vi "05_orezani_signalu_na_celistve_periody.vi"() -> ()   [LabVIEW 2019]
uses:
  <vilib>/Analysis/baseanly.llb/Mean (DBL).vi
  <vilib>/measure/NI_MABase.lvlib
  <vilib>/Analysis/NI_AALBase.lvlib
panel:
  out "Pouze kompletni periody":waveform(dbl)(graph)={"t0"=timestamp(0 s since 1904-01-01), "dt"=0.001, "Y"=array[484 elements]}
  out "Delka signalu celych period":dbl=0.4981312127236578
  out "Pocet celistvych period":dbl=30.0
  out "Necelistvy pocet period?":bool=TRUE
  out "Delka celeho signalu (s)":dbl=0.5
  out "Pocet period":dbl=30.112547892720322
  out "Prumerna perioda signalu(s)":dbl=0.01660437375745526
  out "Prumerna frekvence (Hz)":dbl=60.22509578544064 format="%0.2f"
  in  "Cas necitlivosti (s)":dbl=0.005
  out "Pole casu pruchodu nulou":dbl[](array[numeric])=[0.009000000000000001, 0.017, 0.025, 0.034, 0.042, 0.05, 0.059000000000000004, 0.067, 0.075, 0.084, 0.092, 0.1, 0.109, 0.117, 0.125, 0.134, 0.14200000000000002, 0.15, 0.159, 0.167, 0.17500000000000002, 0.184, 0.192, 0.2, 0.209, 0.217, 0.225, 0.234, 0.242, 0.25, 0.259, 0.267, 0.275, 0.28400000000000003, 0.292, 0.3, 0.309, 0.317, 0.325, 0.334, 0.342, 0.35000000000000003, 0.359, 0.367, 0.375, 0.384, 0.392, 0.4, 0.40900000000000003, 0.417, 0.425, 0.434, 0.442, 0.45, 0.459, 0.467, 0.47500000000000003, 0.484, 0.492]
  out "Originalni signal":waveform(dbl)(graph)={"t0"=timestamp(0 s since 1904-01-01), "dt"=0.001, "Y"=array[500 elements]}
  out "dt (s)":dbl=0.001
  out "Vzorkovaci Frekvence (N)":dbl=1000.0
  in  "Amplituda sumu":dbl format="%.2p"
  in  "Info o vzorkovani":T1={"Vzorkovaci frekvence"=1000.0, "Pocet vzorku v okne"=500.0} {"Vzorkovaci frekvence" format="%.2p"}
  in  "Faze":dbl format="%.2p"
  in  "Amplituda":dbl=10.0 format="%0.2p"
  in  "Frekvence":dbl=60.000000000000604 format="%0.2p"
  # "Jak budete zvedat frekvenci signalu, sledujte, ze mezera mezi nulou a poslednim vzorkem se meni, jelikoz samotna 1 perioda ma\nmene vzorku. Zkuste menit aj vzorkovaci frekvenci."
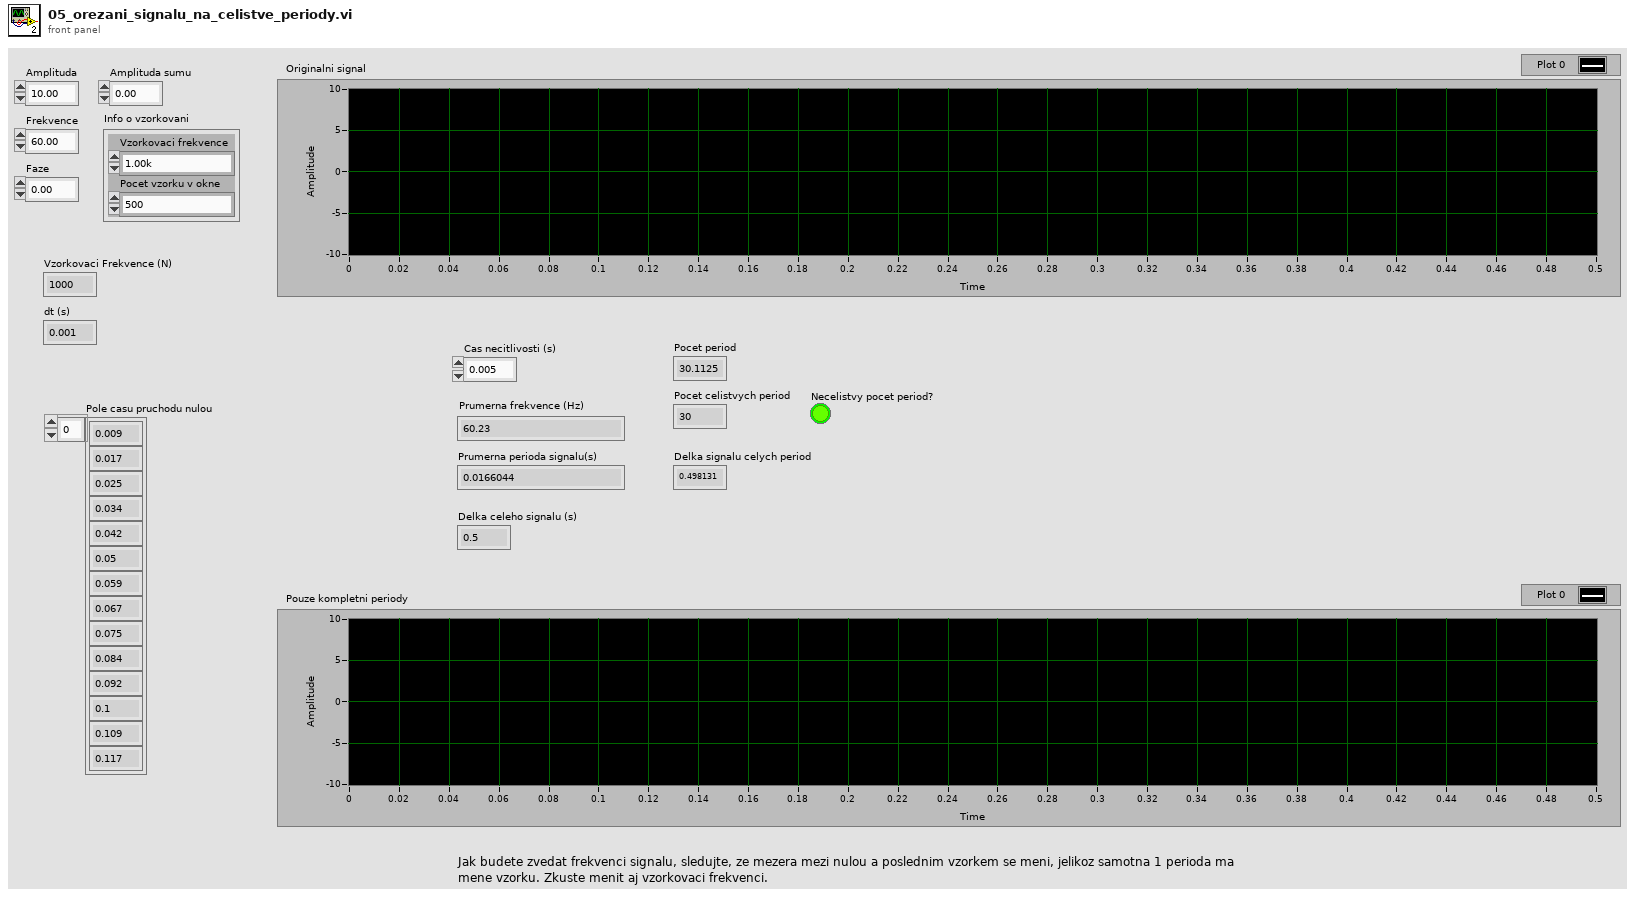
[diagram p1: front panel]
types:
  T1 = cluster{"Vzorkovaci frekvence":dbl, "Pocet vzorku v okne":dbl}
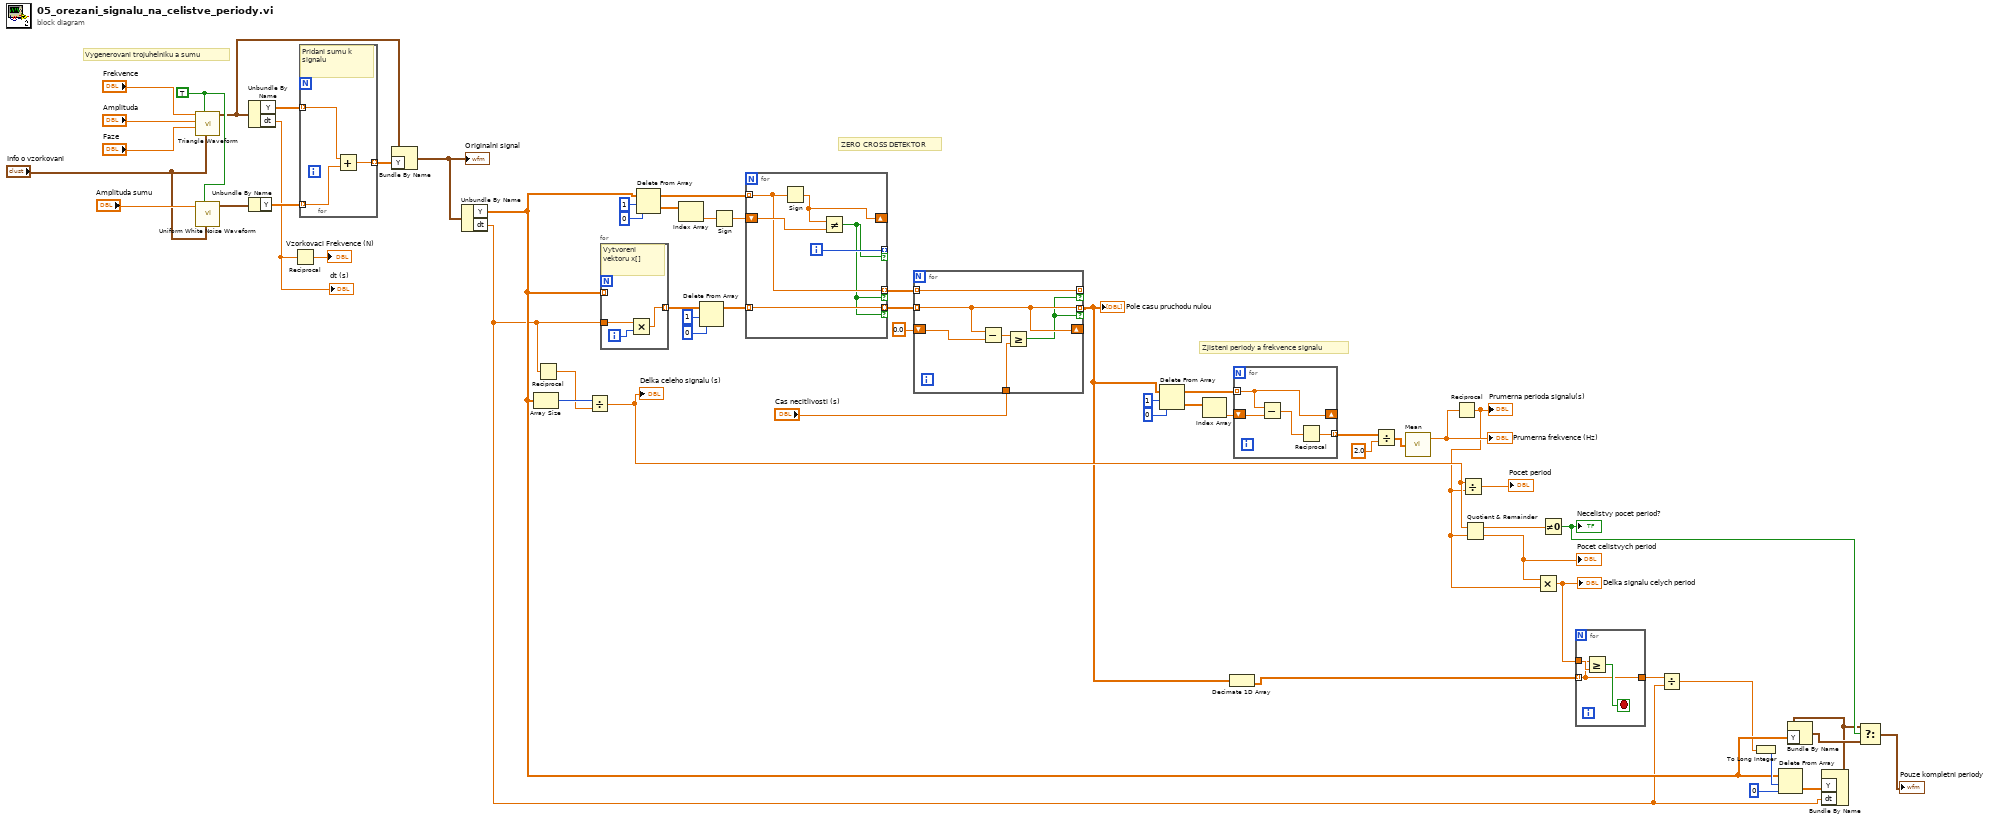
[diagram p0: block diagram]
diagram:
  w54 = TRUE ("reset signal")
  # "Zjisteni periody a frekvence signalu"
  # "ZERO CROSS DETEKTOR"
  # "Vygenerovani trojuhelniku a sumu"
  n1 = call <vilib>:"Triangle Waveform.vi"("sampling info"="Info o vzorkovani", "reset signal"=w54, "phase"="Faze", "amplitude"="Amplituda", "frequency"="Frekvence") -> ("signal out"=w49:waveform(dbl))  [unwired: 5 in, 1 out]
  n2 = call <vilib>:"Uniform White Noise Waveform.vi"("sampling info"="Info o vzorkovani", "reset signal"=w54, "amplitude"="Amplituda sumu") -> ("signal out"=w53:waveform(dbl))  [unwired: 7 in, 1 out]
  n3 = Unbundle By Name(w49) -> ("Y"=w52:dbl[], "dt"=w23:dbl)
  "dt (s)" <- w23
  n4 = Unbundle By Name(w53) -> ("Y"=w51:dbl[])
  n5 = Reciprocal(x=w23) -> (1/x=→"Vzorkovaci Frekvence (N)":dbl)
  n6 = for {
    tunnel: w52 -> [w60] mode=indexing
    tunnel: w51 -> [w61] mode=indexing
    tunnel: [w59] -> w35 mode=indexing
    # "Pridani sumu k signalu"
    n7 = Add(x=w60, y=w61) -> (x+y=w59:dbl)
  }
  n8 = Bundle By Name(cluster=w49, "Y"=w35) -> (w22:waveform(dbl))
  "Originalni signal" <- w22
  n9 = Unbundle By Name(w22) -> ("Y"=w9:dbl[], "dt"=w3:dbl)
  n10 = Array Size(array=w9) -> (size(s)=w21:i32)
  n11 = Reciprocal(x=w3) -> (1/x=w20:dbl)
  n12 = Divide(x=w21, y=w20) -> (x/y=w19:dbl)
  "Delka celeho signalu (s)" <- w19
  n13 = for {
    tunnel: w3 -> [w63]
    tunnel: [w62] -> w41 mode=indexing
    tunnel: w9 -> [_] mode=indexing
    i -> [w64]
    # "Vytvoreni vektoru x[]"
    n14 = Multiply(x=w63, y=w64) -> (x*y=w62:dbl)
  }
  n15 = Delete From Array(array=w9, length=1, index=0) -> (deleted portion=w45:dbl[], array with subset deleted=w48:dbl[])
  n16 = Index Array(array=w45) -> (element=w40:dbl)  [unwired: 1 in]
  n17 = Delete From Array(array=w41, length=1, index=0) -> (array with subset deleted=w42:dbl[])  [unwired: 1 out]
  n18 = Sign(1:w40) -> (0:w39:dbl)
  n19 = for {
    tunnel: w48 -> [w66] mode=indexing
    shift-right: [w70] -> _
    shift-left: w39 -> [w69]
    tunnel: [w68] -> _ mode=indexing if=w65
    tunnel: w42 -> [w67] mode=indexing
    tunnel: [w67] -> w38 mode=indexing if=w65
    tunnel: [w66] -> w36 mode=indexing if=w65
    i -> [w68]
    # "Detekce pruchodu nulou"
    n20 = Sign(1:w66) -> (0:w70:dbl)
    n21 = Not Equal?(x=w70, y=w69) -> (x != y?=w65:bool)
  }
  n22 = for {
    tunnel: w38 -> [w74] mode=indexing
    shift-right: [w74] -> _
    shift-left: 0.0 -> [w75]
    tunnel: [w74] -> w6 mode=indexing if=w72
    tunnel: w36 -> [w73] mode=indexing
    tunnel: [w73] -> _ mode=indexing if=w72
    tunnel: "Cas necitlivosti (s)" -> [w71]
    # "Oproti predchozimu pristupu o mnoho lepsi. Nezahazujeme kazdy druhy vzorek ale jen ty ktere nesplnuji podminku a jsou v pasmu necitlivosti"
    n23 = Subtract(x=w74, y=w75) -> (x-y=w76:dbl)
    n24 = Greater Or Equal?(x=w76, y=w71) -> (x >= y?=w72:bool)
  }
  "Pole casu pruchodu nulou" <- w6
  n25 = Delete From Array(array=w6, length=1, index=0) -> (deleted portion=w33:dbl[], array with subset deleted=w30:dbl[])
  n26 = Index Array(array=w33) -> (element=w29:dbl)  [unwired: 1 in]
  n27 = Decimate 1D Array(w6) -> (w1:dbl[])  [unwired: 1 out]
  n28 = for {
    tunnel: w30 -> [w80] mode=indexing
    shift-right: [w80] -> _
    shift-left: w29 -> [w79]
    tunnel: [w77] -> w28 mode=indexing
    # "Prepocet absolutnich casovych hodnot na vzajemne relativni vzdalenosti jednotlivych pruchodu nulou => vzdalenost dvou puntiku od sebe"
    n29 = Subtract(x=w80, y=w79) -> (x-y=w78:dbl)
    n30 = Reciprocal(x=w78) -> (1/x=w77:dbl)
  }
  n31 = Divide(x=w28, y=2.0) -> (x/y=w26:dbl[])
  n32 = call-poly <vilib>:"Mean.vi"("X"=w26) -> ("mean"=w25:dbl)  [unwired: 1 out]
  "Prumerna frekvence (Hz)" <- w25
  n33 = Reciprocal(x=w25) -> (1/x=w15:dbl)
  "Prumerna perioda signalu(s)" <- w15
  n34 = Divide(x=w19, y=w15) -> (x/y=→"Pocet period":dbl)
  n35 = Quotient & Remainder(x=w19, y=w15) -> (x-y*floor(x/y)=w17:dbl, floor(x/y)=w16:dbl)
  "Pocet celistvych period" <- w16
  n36 = Multiply(x=w16, y=w15) -> (x*y=w5:dbl)
  "Delka signalu celych period" <- w5
  n37 = Not Equal To 0?(x=w17) -> (x != 0?=w11:bool)
  "Necelistvy pocet period?" <- w11
  n38 = for {
    tunnel: w1 -> [w81] mode=indexing
    tunnel: w5 -> [w83]
    tunnel: [w81] -> w4
    stop <- w82 stop-if-true
    n39 = Greater Or Equal?(x=w81, y=w83) -> (x >= y?=w82:bool)
  }
  n40 = Divide(x=w4, y=w3) -> (x/y=w2:dbl)
  n41 = To Long Integer(number=w2) -> (32bit integer=w14:i32)
  n42 = Delete From Array(array=w9, length=w14, index=0) -> (deleted portion=w12:dbl[])  [unwired: 1 out]
  n43 = Bundle By Name("Y"=w12, "dt"=w3) -> (w7:waveform(dbl))  [unwired: 1 in]
  n44 = Bundle By Name(cluster=w7, "Y"=w9) -> (w8:waveform(dbl))
  n45 = Select(t=w7, s=w11, f=w8) -> (s? t:f=→"Pouze kompletni periody":waveform(dbl))
